vi "Pie Chart customized.vi"() -> (3 "Picture":picture)   [LabVIEW 2016, in "CML UI.lvlib" / "Circular Cue Helper.lvlib"]
doc: "This VI generates a pie chart using the LabVIEW picture control. Given an array of clusters containing a label and a value, a pie chart with legend is generated and displayed."
uses:
  Circular Cue Helper.lvlib
  <vilib>/Utility/miscctls.llb/LVBoundsTypeDef.ctl
panel:
  out "Delay":dbl
  in  "Input":cluster{"Label":string, "Value":dbl}[](array[cluster])=[{"Label"="This", "Value"=23.0}, {"Label"="is", "Value"=13.0}, {"Label"="only", "Value"=36.0}, {"Label"="a", "Value"=7.0}, {"Label"="test", "Value"=21.0}]
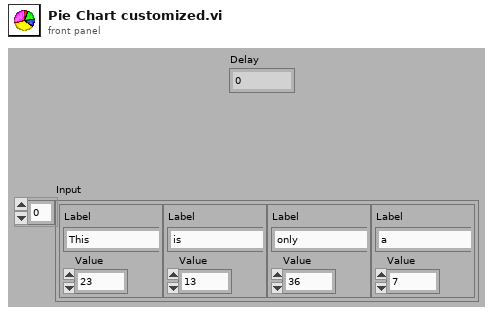
[diagram p1: front panel]
types:
  T1 = cluster{"left":i16, "top":i16, "right":i16, "bottom":i16}
  T2 = typedef "LVBoundsTypeDef.ctl" = cluster{"Width":u32, "Height":u32}
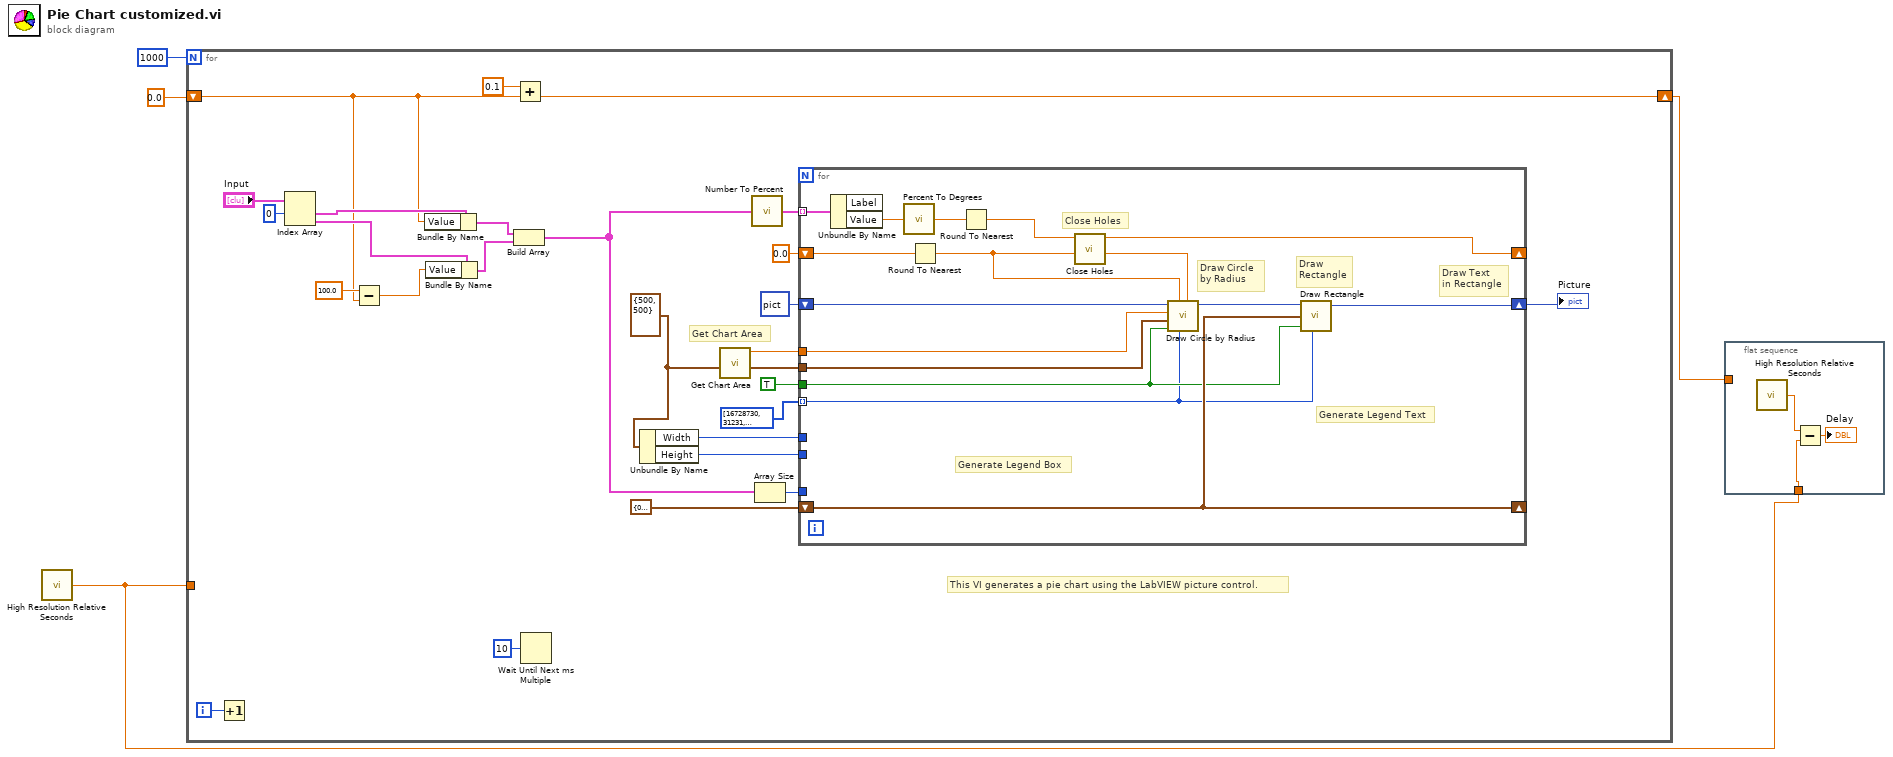
[diagram p0: block diagram]
diagram:
  n1 = call <vilib>:"High Resolution Relative Seconds.vi"() -> ("relative seconds"=w1:dbl)
  n2 = for {
    N: 1000 -> [_]
    shift-right: [w9] -> w2
    shift-left: 0.0 -> [w6]
    tunnel: w1 -> [_]
    i -> [w10]
    w20 = T2 {"Width"=500, "Height"=500} ("Draw Area Size")
    # "This VI generates a pie chart using the LabVIEW picture control."
    # "Get Chart Area"
    n3 = Increment(x=w10) -> ()  [unwired: 1 out]
    n4 = Index Array(array="Input", index #1=0 ("index")) -> (element #1=w16:cluster{"Label":string, "Value":dbl}, element #2=w15:cluster{"Label":string, "Value":dbl})  [unwired: 1 in]
    n5 = Subtract(x=100.0, y=w6) -> (x-y=w5:dbl)
    n6 = Bundle By Name(cluster=w16, "Value"=w6) -> (w14:cluster{"Label":string, "Value":dbl})
    n7 = Bundle By Name(cluster=w15, "Value"=w5) -> (w13:cluster{"Label":string, "Value":dbl})
    n8 = Build Array(w14, w13) -> (w12:cluster{"Label":string, "Value":dbl}[])
    n9 = Add(x=0.1, y=w6) -> (x+y=w9:dbl)
    n10 = Wait Until Next ms Multiple(millisecond multiple=u32 10) -> ()  [unwired: 1 out]
    n11 = Unbundle By Name(w20) -> ("Width"=w26:u32, "Height"=w28:u32)
    n12 = call "Get Chart Area.vi"("Draw Area Size"=w20) -> ("Chart Area Size"=w19:cluster{"Width":dbl, "Height":dbl}, "Height"=w21:dbl)  [unwired: 9 in]
    n13 = call "Number To Percent.vi"("Array In"=w12) -> ("Array Out"=w23:cluster{"Label":string, "Value":dbl}[])
    n14 = Array Size(array=w12) -> (size(s)=w22:i32)
    n15 = for {
      tunnel: w23 -> [w47] mode=indexing
      shift-right: [w40] -> w29
      shift-left: picture data[5B] ("new picture") -> [w46]
      tunnel: w21 -> [w42]
      shift-right: [w34] -> _
      shift-left: 0.0 -> [w38]
      tunnel: u32[] [16728730, 31231, 327900, 441827, 16512, 2768895, 11121611, 7171459, 0] -> [w39] mode=indexing
      shift-right: [w43] -> _
      shift-left: T1 {"left"=0, "top"=0, "right"=0, "bottom"=0} ("rect") -> [w43]
      tunnel: w28 -> [_]
      tunnel: TRUE ("fill?(F)") -> [w41]
      tunnel: w26 -> [_]
      tunnel: w22 -> [_]
      tunnel: w19 -> [w32]
      # "Draw Circle \nby Radius"
      # "Draw Text\nin Rectangle"
      # "Draw \nRectangle"
      # "Close Holes"
      # "Generate Legend Text"
      # "Generate Legend Box"
      n16 = Unbundle By Name(w47) -> ("Value"=w45:dbl)  [unwired: 1 out]
      n17 = call "Percent To Degrees.vi"("Percent"=w45) -> ("Degrees"=w36:dbl)
      n18 = Round To Nearest(number=w38) -> (nearest integer value=w37:dbl)
      n19 = Round To Nearest(number=w36) -> (nearest integer value=w33:dbl)
      n20 = call "Close Holes.vi"("Start Angle"=w37, "Preliminary Arc Size"=w33) -> ("Final Arc Size"=w35:dbl, "Final Angle"=w34:dbl)  [unwired: 8 out]
      n21 = call <vilib>:"Draw Circle by Radius.vi"("arc size(360)"=w35, "color(black)"=w39, "start angle(0)"=w37, "fill?(F)"=w41, "pixel center"=w32, "radius"=w42, "picture"=w46) -> ("new picture"=w44:picture)  [unwired: 1 in, 3 out]
      n22 = call <vilib>:"Draw Rectangle.vi"("picture"=w44, "rect"=w43, "fill?(F)"=w41, "color(black)"=w39) -> ("new picture"=w40:picture)  [unwired: 5 in]
    }
    "Picture" <- w29
  }
  n23 = flat-sequence {
    tunnel: w2 -> [_]
    tunnel: w1 -> [w49]
    frame #0 {
      n24 = call <vilib>:"High Resolution Relative Seconds.vi"() -> ("relative seconds"=w50:dbl)
      n25 = Subtract(x=w50, y=w49) -> (x-y=→"Delay":dbl)
    }
  }
